vi "ED_Close.vi"(4 "error in (no error)":errorcluster, 7 "connection ID":refnum<k5>) -> (0 "error out":errorcluster)   [LabVIEW 2013, in "CAENels EASY-DRIVER.lvlib"]
doc: "Closes the connection."
uses:
  CAENels EASY-DRIVER.lvlib
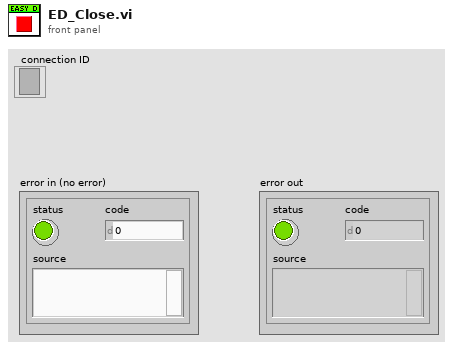
[diagram p1: front panel]
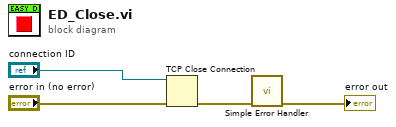
[diagram p0: block diagram]
diagram:
  n1 = TCP Close Connection(connection ID="connection ID", error in (no error)="error in (no error)") -> (error out=w2:errorcluster)  [unwired: 1 in, 1 out]
  n2 = call "Simple Error Handler.vi"("error in (no error)"=w2) -> ("error out"=→"error out":errorcluster)  [unwired: 4 in, 4 out]
